vi "Do.vi"(8 "error in (no error)":errorcluster, 10 "Actor in":refnum<class "Actor.lvclass">, 11 "Record Trace Msg":refnum<class "Record Trace Msg.lvclass">) -> (0 "error out":errorcluster, 2 "Actor out":refnum<class "Actor.lvclass">)   [LabVIEW 2014, in "Robot Actor Framework.lvlib" / "System Actor.lvlib" / "Record Trace Msg.lvclass"]
doc: "This VI delivers the message to the actor by calling the appropriate method(s) on the actor."
uses:
  Record Trace Msg.lvclass
  <vilib>/ActorFramework/Actor/Actor.lvclass
  Record Trace Msg.lvclass/Record Trace Msg.ctl
  System Actor Class/System Actor.lvclass
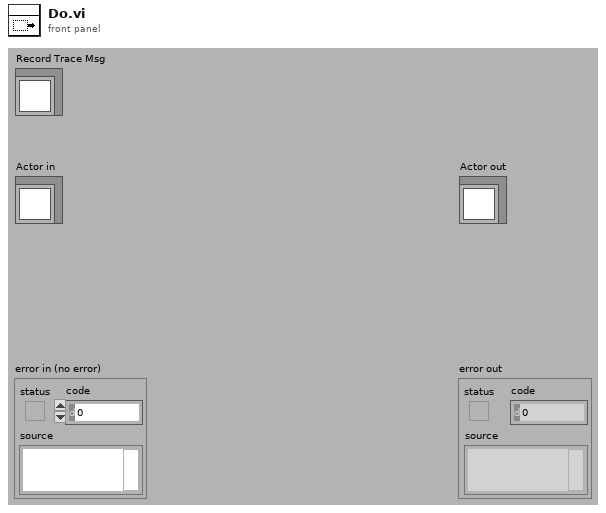
[diagram p1: front panel]
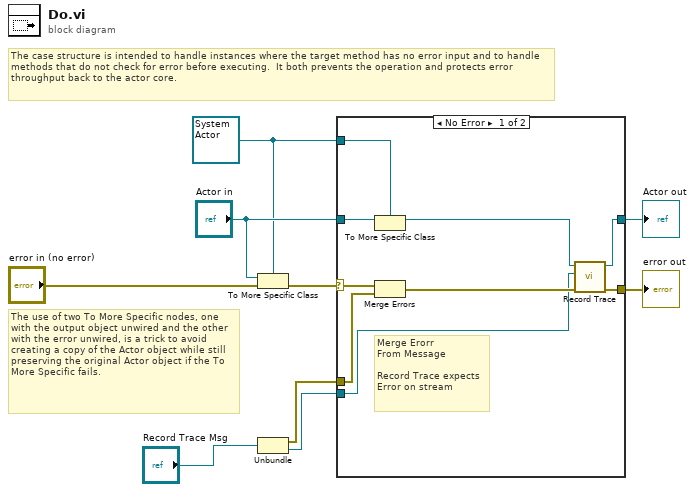
[diagram p0: block diagram]
diagram:
  w3 = refnum<class "System Actor.lvclass"> refnum ("Actor in")
  # "The use of two To More Specific nodes, one with the output object unwired and the other with the error unwired, is a trick to avoid creating a copy of the Actor object while still preserving the original Actor object if the To More Specific fails."
  # "The case structure is intended to handle instances where the target method has no error input and to handle methods that do not check for error before executing.  It both prevents the operation and protects error throughput back to the actor core."
  n1 = To More Specific Class(target class=w3, reference="Actor in", error in="error in (no error)") -> (error out=w7:errorcluster)  [unwired: 1 out]
  n2 = Unbundle("Record Trace Msg") -> (w2:errorcluster, w1:refnum<class "Trace.lvclass">)
  n3 = case shown="No Error" w7 {
    selector: w7 -> [w16 w20]
    tunnel: [w18 w20] -> w6
    tunnel: [w17 w19] -> w5
    tunnel: "Actor in" -> [w15 w19]
    tunnel: w3 -> [w14 _]
    tunnel: w2 -> [w10 _]
    tunnel: w1 -> [w11 _]
    frame No Error {
      # "Merge Erorr \nFrom Message\n\nRecord Trace expects\nError on stream"
      n4 = To More Specific Class(target class=w14, reference=w15) -> (specific class reference=w13:refnum<class "System Actor.lvclass">)  [unwired: 1 in, 1 out]
      n5 = Merge Errors(w16, w10) -> (w12:errorcluster)
      n6 = call-dynamic "Record Trace.vi"("error in (no error)"=w12, "Trace"=w11, "System Actor in"=w13) -> ("error out"=w18:errorcluster, "System Actor out"=w17:refnum<class "System Actor.lvclass">)  [unwired: 7 in]
    }
    frame Error {
      # "If type check fails, pass the original object out again."
    }
  }
  "error out" <- w6
  "Actor out" <- w5
